vi "App Strings.vi"() -> ()   [LabVIEW 2015]
panel:
  in  "Error msg":string
  in  "Acq Error":string="Nie udało się ukończyć pomiaru w zdefiniowanym czasie"
  in  "Acq Finished":string="Pomiar zakończył się sukcesem"
  in  "Acq Start":string="Pomiar trwa........."
  # "#Obserwacja \nCzęsto w aplikacjach, które piszemy umieszczamy teksty komunikatów w zmiennej globalnej. Dzięki temu wyglądają one tak samo w kożdym miejscu i nie musimy w kodzie wpisywać stałej zawierającej bardzo długi tekst, wystaczy wybrać nazwę kontrolki.\nZamiast pisania \"Nie udało się ukończyć pomiaru w zdefiniowanym czasie\" wybieramy Acq Error\n\nPamiętaj o wybraniu opcji Edit/ Make current Values Default"
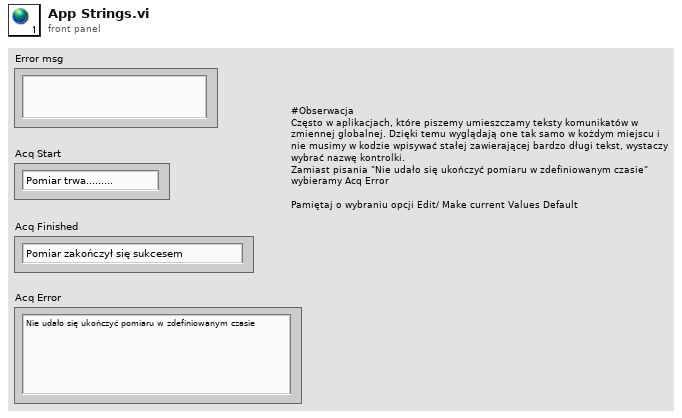
[diagram p1: front panel]
diagram:
